vi "pf_Error_builder.vi"(7 "pf Error Type":T1, 11 "Error message":string) -> (0 "Error cluster out":errorcluster)   [LabVIEW 2025, in "Photonfocus_Toolkit.lvlib"]
uses:
  Photonfocus_Toolkit.lvlib
  Controls/pf_Toolkit_Error_Type.ctl
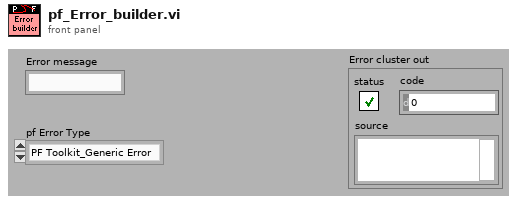
[diagram p1: front panel]
types:
  T1 = typedef "Photonfocus_Toolkit.lvlib/pf_Toolkit_Error_Type.ctl" = enum16{"PF Toolkit_Generic Error", "PF Toolkit_PFConfig Error"}
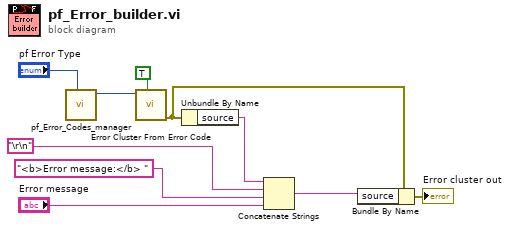
[diagram p0: block diagram]
diagram:
  n1 = call "pf_Error_Codes_manager.vi"("pf Error Type"="pf Error Type") -> ("pf Error Code"=w8:i32)  [unwired: 1 in, 9 out]
  n2 = call <vilib>:"Error Cluster From Error Code.vi"("show call chain? (False)"=TRUE, "error code (0)"=w8) -> ("error out"=w1:errorcluster)  [unwired: 1 in, 6 out]
  n3 = Unbundle By Name(w1) -> ("source"=w7:string)
  n4 = Concatenate Strings(w7, "\r\n", "<b>Error message:</b> " ("string"), "Error message") -> (w5:string)
  n5 = Bundle By Name(cluster=w1, "source"=w5) -> (→"Error cluster out":errorcluster)
